vi "Add Packages to a Feed.vi"() -> ()   [LabVIEW 2014]
doc: "This example shows how to add packages to a feed. This example also gives the user the option of creating a new feed in the specified feed folderpath, if necessary."
uses:
  NIPM_API.lvlib
panel:
  in  "Add package":bool
  out "Package names and versions in this feed":string[][](array[string])
  in  "package (.nipkg) source filepath":path
  out "Feed created?":bool
  in  "Create new feed in folder (if necessary)":bool
  in  "feed folderpath":path
  # "Feed Information"
  # "Package to add to the feed"
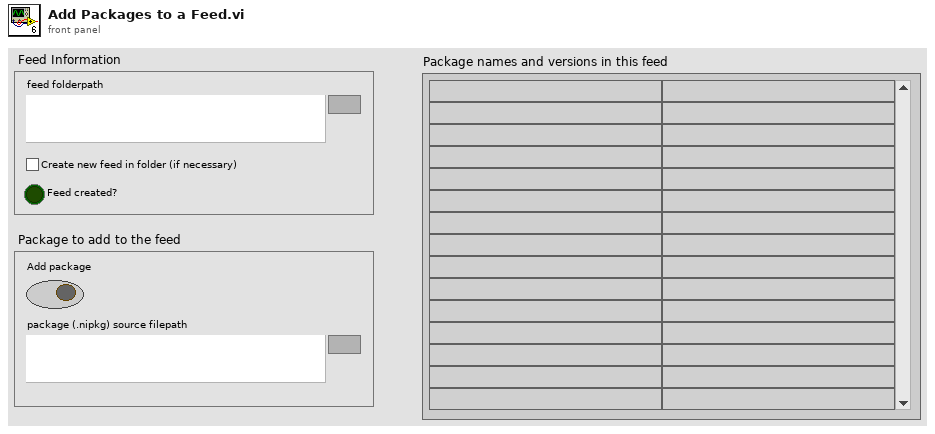
[diagram p1: front panel]
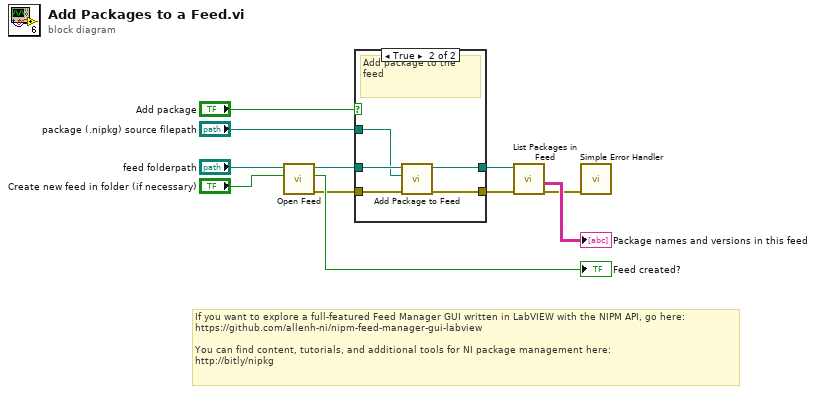
[diagram p0: block diagram]
diagram:
  # "If you want to explore a full-featured Feed Manager GUI written in LabVIEW with the NIPM API, go here:\nhttps://github.com/allenh-ni/nipm-feed-manager-gui-labview\n\nYou can find content, tutorials, and additional tools for NI package management here:\nhttp://bitly/nipkg"
  n1 = call "Open Feed.vi"("create feed if necessary (F)"="Create new feed in folder (if necessary)", "feed folderpath"="feed folderpath") -> ("error out"=w8:errorcluster, "feed created?"=→"Feed created?":bool, "feed folderpath out"=w5:path)  [unwired: 7 in]
  n2 = case shown="True" "Add package" {
    tunnel: w8 -> [w12 w18]
    tunnel: [w12 w17] -> w6
    tunnel: w5 -> [w13 w16]
    tunnel: [w13 w15] -> w4
    tunnel: "package (.nipkg) source filepath" -> [_ w14]
    frame False {
      # "Don't add package to the feed"
    }
    frame True {
      # "Add package to the feed"
      n3 = call "Add Package to Feed.vi"("error in"=w18, "package source filepath"=w14, "feed folderpath in"=w16) -> ("error out"=w17:errorcluster, "feed folderpath out"=w15:path)  [unwired: 6 in, 1 out]
    }
  }
  n4 = call "List Packages in Feed.vi"("error in"=w6, "feed folderpath in"=w4) -> ("error out"=w2:errorcluster, "package names and versions"=→"Package names and versions in this feed":string[][])  [unwired: 6 in, 2 out]
  n5 = call <vilib>:"Simple Error Handler.vi"("error in (no error)"=w2) -> ()  [unwired: 4 in, 5 out]
